vi "Move.vi"(8 "error in (no error)":errorcluster, 11 "Snake in":refnum<class "Snake.lvclass">) -> (0 "error out":errorcluster, 3 "Snake out":refnum<class "Snake.lvclass">)   [LabVIEW 2021, in "Snake.lvclass"]
uses:
  Snake.lvclass
  Snake.lvclass/Snake.ctl
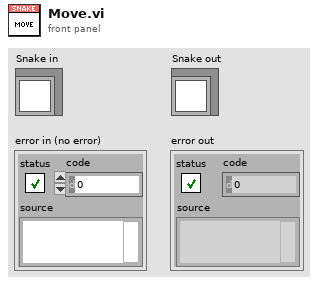
[diagram p1: front panel]
types:
  T1 = typedef "Position.ctl" = cluster{"X":i32, "Y":i32}
  T2 = typedef "Direction.ctl" = enum16{"Up", "Down", "Left", "Right"}
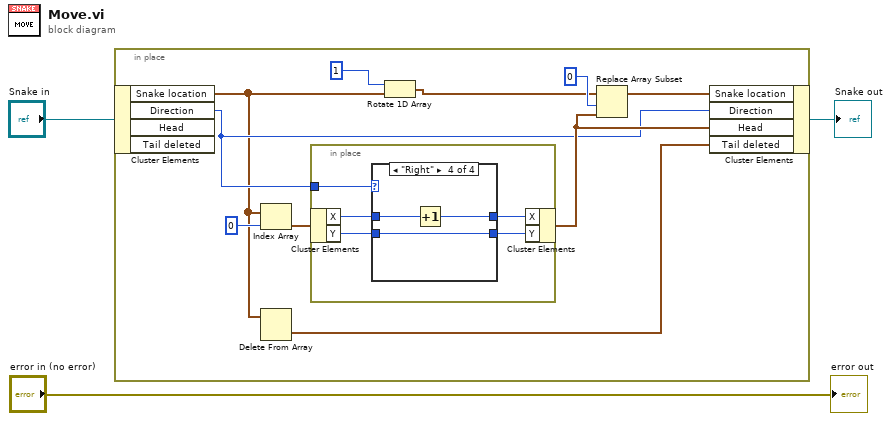
[diagram p0: block diagram]
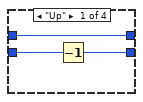
[diagram p2: hidden frame]
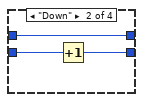
[diagram p3: hidden frame]
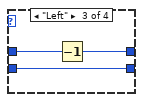
[diagram p4: hidden frame]
diagram:
  n1 = in-place {
    n2 = in-place-cluster #1("Snake in") -> ("Snake location"=w5:T1[], "Direction"=w8:T2)  [unwired: 2 out]
    n3 = Index Array(array=w5, index=0) -> (element=w10:T1)
    n4 = Delete From Array(array=w5) -> (deleted portion=w6:T1)  [unwired: 2 in, 1 out]
    n5 = in-place {
      in-place-border: w8 -> [w18]
      n6 = in-place-cluster #2(w10) -> ("X"=w17:i32, "Y"=w16:i32)
      n7 = case shown="\"Right\"" w18 {
        tunnel: w17 -> [w21 w24 w27 w30]
        tunnel: w16 -> [w20 w23 w26 w29]
        tunnel: [w21 w24 w25 w28] -> w15
        tunnel: [w19 w22 w26 w29] -> w14
        frame "Up" {
          n8 = Decrement(x=w20) -> (x-1=w19:i32)
        }
        frame "Down" {
          n9 = Increment(x=w23) -> (x+1=w22:i32)
        }
        frame "Left" {
          n10 = Decrement(x=w27) -> (x-1=w25:i32)
        }
        frame "Right" {
          n11 = Increment(x=w30) -> (x+1=w28:i32)
        }
      }
      n12 = in-place-cluster #2("X"=w15, "Y"=w14) -> (w9:T1)
    }
    n13 = Rotate 1D Array(1:w5, 2:1 ("n")) -> (0:w4:T1[])
    n14 = Replace Array Subset "Replace Array Subset"(array=w4, new element=w9, index=0) -> (w12:T1[])
    n15 = in-place-cluster #1("Snake location"=w12, "Direction"=w8, "Head"=w9, "Tail deleted"=w6) -> (→"Snake out":refnum<class "Snake.lvclass">)
  }
  "error out" <- "error in (no error)"
